vi "List Tables.vi"(8 "error in (no error)":errorcluster, 10 "Database in":string, 11 "sqlite in":refnum<class "sqlite3.lvclass">) -> (0 "error out":errorcluster, 2 "Tables out":string[](array[string]), 3 "sqlite out":refnum<class "sqlite3.lvclass">)   [LabVIEW 2020, in "sqlite3.lvlib" / "sqlite3.lvclass"]
uses:
  sqlite3.lvclass
  sqlite3.lvclass/sqlite3.ctl
  db layer/compound/Execute SQL.vi
  <vilib>/Utility/error.llb/Clear Errors.vi
  sqlite/VIs/open v2.vi
  sqlite/VIs/prepare v2.vi
  sqlite/VIs/step.vi
  sqlite/VIs/column count.vi
  db layer/compound/Column.vi
  db layer/compound/Resolve Result Type.vi
  sqlite/VIs/finalize.vi
  sqlite/VIs/close v2.vi
  sqlite/subvi/Error Converter (ErrCode or Status).vi
  sqlite/VIs/column text.vi
  sqlite/VIs/column bytes.vi
  sqlite/VIs/column blob.vi
  db layer/utilities/MoveBlock.vi
  sqlite/VIs/column type.vi
  sqlite/VIs/errstr.vi
  sqlite3.lvlib
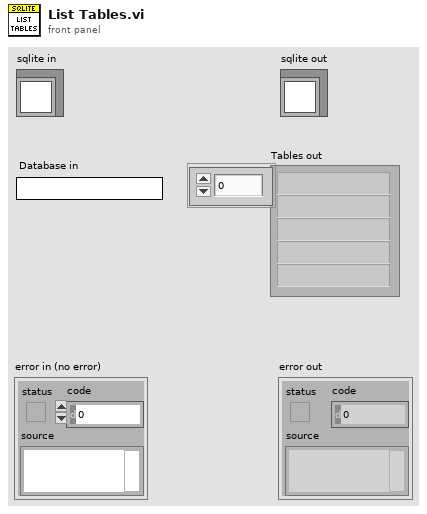
[diagram p1: front panel]
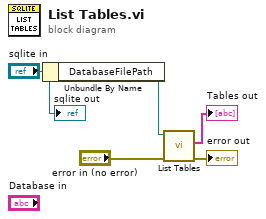
[diagram p0: block diagram]
diagram:
  n1 = Unbundle By Name("sqlite in") -> ("DatabaseFilePath"=w4:path)
  n2 = call "List Tables.vi"("error in (no error)"="error in (no error)", "database in"=w4) -> ("error out"=→"error out":errorcluster, "Tables"=→"Tables out":string[])  [unwired: 8 in]
  "sqlite out" <- "sqlite in"
